vi "SetAllVisibleGraphCtrl.vi"(7 "plot count":i32, 10 "on/off":bool, 11 "ref graph in":refnum<vi>) -> (3 "ref graph out":refnum<vi>)   [LabVIEW 2018, in "Library-Ctrl.lvlib"]
uses:
  Library-Ctrl.lvlib
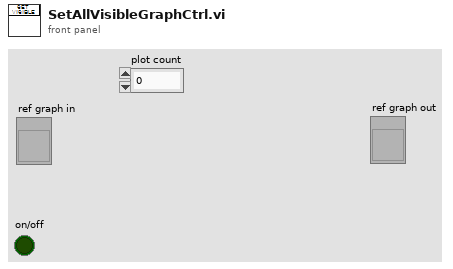
[diagram p1: front panel]
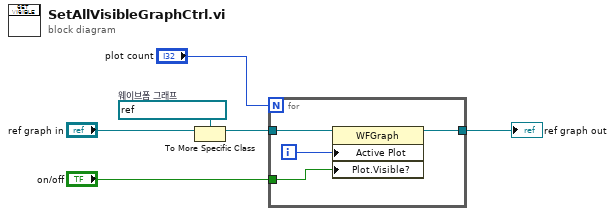
[diagram p0: block diagram]
diagram:
  w5 = refnum<vi> refnum  # 웨이브폼 그래프
  n1 = To More Specific Class(target class=w5, reference="ref graph in") -> (specific class reference=w4:refnum<vi>)  [unwired: 1 in, 1 out]
  n2 = for {
    N: "plot count" -> [_]
    tunnel: w4 -> [w10]
    tunnel: [w8] -> w2
    tunnel: "on/off" -> [w7]
    i -> [w9]
    n3 = property class="WFGraph"(reference=w10, "Active Plot"=w9, "Plot.Visible?"=w7) -> (reference out=w8:refnum<vi>)  [unwired: 1 in, 1 out]
  }
  "ref graph out" <- w2
